vi "Problem1.8a-RandomNumber-SubVI.vi"() -> (0 "Uniform Deviate":dbl, 3 "Initial Random Number":dbl)   [LabVIEW 2019]
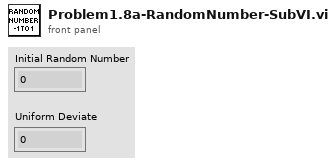
[diagram p1: front panel]
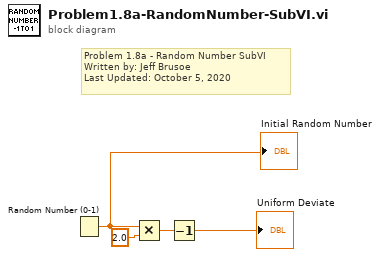
[diagram p0: block diagram]
diagram:
  # "Problem 1.8a - Random Number SubVI\nWritten by: Jeff Brusoe\nLast Updated: October 5, 2020"
  n1 = Random Number (0-1)() -> (number: 0 to 1=w4:dbl)
  "Initial Random Number" <- w4
  n2 = Multiply(x=w4, y=2.0) -> (x*y=w2:dbl)
  n3 = Decrement(x=w2) -> (x-1=→"Uniform Deviate":dbl)
